vi "Get Config File Path.vi"(11 "Model Name":string) -> (3 "appended path":path)   [LabVIEW 2025, in "PLC_Module.lvlib" / "PLC_Module.lvclass"]
uses:
  PLC_Module.lvclass
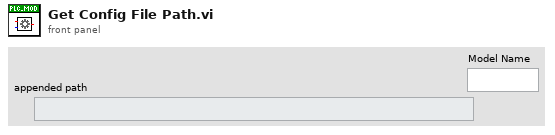
[diagram p1: front panel]
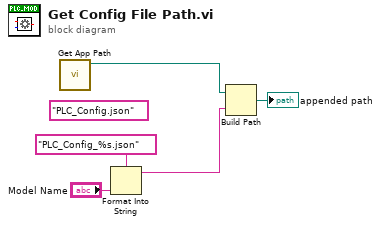
[diagram p0: block diagram]
diagram:
  (unwired) "PLC_Config.json"
  n1 = call "Get App Path.vi"() -> ("Parent Directory (+ Relative)"=w4:path)  [unwired: 11 in]
  n2 = Format Into String(format string="PLC_Config_%s.json", "Model Name") -> (resulting string=w2:string)  [unwired: 2 in, 1 out]
  n3 = Build Path(base path=w4, name or relative path=w2) -> (appended path=→"appended path":path)
